vi "CalibratedGratingv1 (obsolite).vi"() -> ()   [LabVIEW 2019]
panel:
  in  "Calibration constant":dbl=1889.0 format="%#_13g"
  in  "Laser:":u16(ring) items=["800nm  "]
  out "Position on spectrometer (pixels):":dbl
  in  "?":bool
  out "Highest Harmonic:":dbl
  out "Lowest Harmonic:":dbl
  out "Beta2 (deg):":dbl
  out "Beta1 (deg):":dbl
  in  "Grating:":u16(ring) items=["Shimadzu 30-006  "]
  out "Anglular position of peak (deg):":dbl
  in  "Harmonic":dbl min=10.0 max=40.0
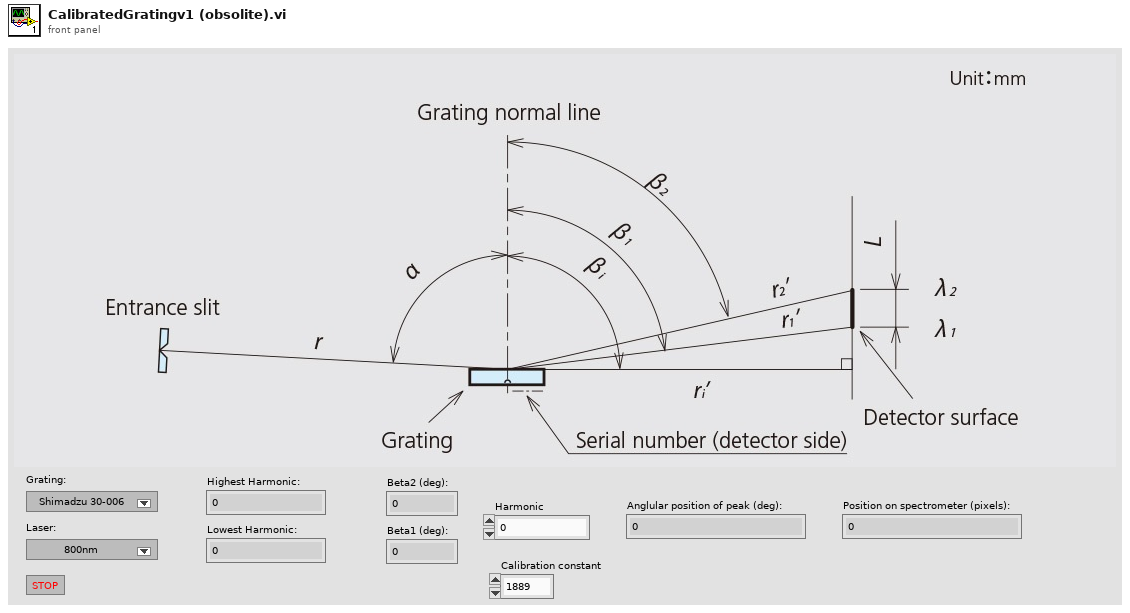
[diagram p1: front panel]
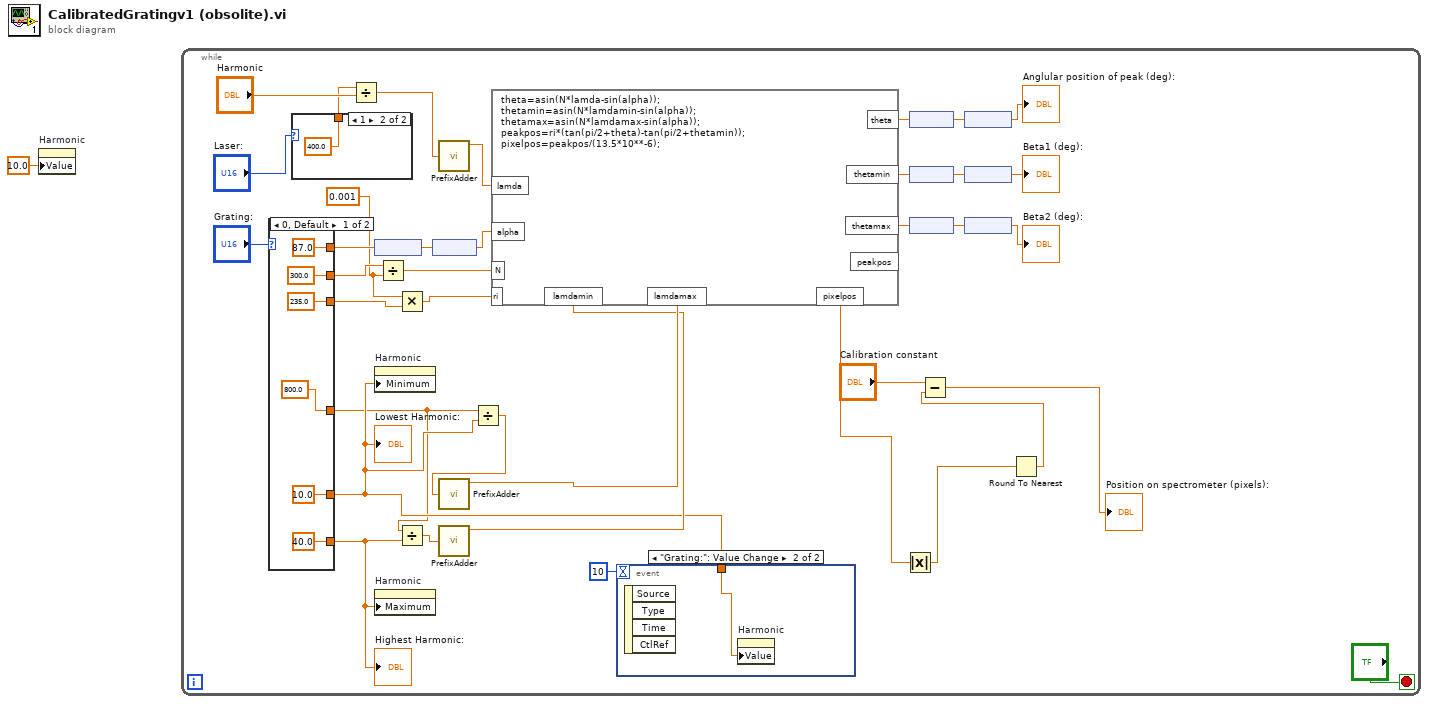
[diagram p0: block diagram]
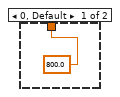
[diagram p2: hidden frame]
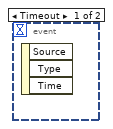
[diagram p3: hidden frame]
diagram:
  n1 = property on="Harmonic" class="DigNum (strict)"("Value"=10.0 ("Wavelegnth (nm)")) -> ()  [unwired: 2 in, 2 out]
  n2 = while {
    stop <- "?" stop-if-true
    w19 = 0.001 ("y")
    n3 = case shown="0, Default" "Grating:" {
      tunnel: [300.0 _] -> w35
      tunnel: [87.0 _] -> w34
      tunnel: [10.0 _] -> w8
      tunnel: [40.0 _] -> w9
      tunnel: [235.0 _] -> w21
      tunnel: [800.0 _] -> w2
      frame 0, Default {
      }
      frame 1 {
      }
    }
    "Lowest Harmonic:" <- w8
    "Highest Harmonic:" <- w9
    n4 = case shown="1" "Laser:" {
      tunnel: [800.0 400.0] -> w3
      frame 0, Default {
      }
      frame 1 {
      }
    }
    n5 = Divide(x=w3, y="Harmonic") -> (x/y=w16:dbl)
    n6 = node(w34) -> (w33:dbl[unit])
    n7 = property on="Harmonic" class="DigNum (strict)"("Minimum"=w8) -> ()  [unwired: 2 in, 2 out]
    n8 = property on="Harmonic" class="DigNum (strict)"("Maximum"=w9) -> ()  [unwired: 2 in, 2 out]
    n9 = Divide(x=w35, y=w19) -> (x/y=w36:dbl)
    n10 = Multiply(x=w19, y=w21) -> (x*y=w20:dbl)
    n11 = Divide(x=w2, y=w9) -> (x/y=w11:dbl)
    n12 = node(w33) -> (w32:dbl)
    n13 = call "PrefixAdder.vi"("No prefix"=w16) -> ("Nano"=w37:dbl)  [unwired: 3 out]
    n14 = call "PrefixAdder.vi"("No prefix"=w11) -> ("Nano"=w12:dbl)  [unwired: 3 out]
    n15 = Divide(x=w2, y=w8) -> (x/y=w10:dbl)
    n16 = call "PrefixAdder.vi"("No prefix"=w10) -> ("Nano"=w13:dbl)  [unwired: 3 out]
    n17 = formula code="theta=asin(N*lamda-sin(alpha));\nthetamin=asin(N*lamdamin-sin(alpha));\nthetamax=asin(N*lamdamax-sin(alpha));\npeakpos=ri*(tan(pi/2+theta)-tan(pi/2+thetamin));\npixelpos=peakpos/(13.5*10**-6);"("lamda"=w37, "N"=w36, "alpha"=w32, "lamdamin"=w12, "lamdamax"=w13, "ri"=w20) -> ("theta"=w22:dbl, "thetamin"=w26:dbl, "thetamax"=w27:dbl, "pixelpos"=w14:dbl)  [unwired: 1 out]
    n18 = event shown="[1] \"Grating:\": Value Change" {
      selector: _ -> [_ _]
      dyn-events: _ -> [_ _]
      timeout: 10 -> [_ _]
      tunnel: w8 -> [_ w41]
      event Timeout {
        n19 = event-data() -> ()  [unwired: 1 in, 3 out]
      }
      event "Grating:": Value Change {
        n20 = event-data() -> ()  [unwired: 1 in, 4 out]
        n21 = property on="Harmonic" class="DigNum (strict)"("Value"=w41) -> ()  [unwired: 2 in, 2 out]
      }
    }
    n22 = Absolute Value(x=w14) -> (abs(x)=w5:dbl)
    n23 = node(w22) -> (w31:dbl[unit])
    n24 = node(w26) -> (w29:dbl[unit])
    n25 = node(w27) -> (w28:dbl[unit])
    n26 = node(w31) -> (→"Anglular position of peak (deg):":dbl)
    n27 = node(w29) -> (→"Beta1 (deg):":dbl)
    n28 = node(w28) -> (→"Beta2 (deg):":dbl)
    n29 = Round To Nearest(number=w5) -> (nearest integer value=w4:dbl)
    n30 = Subtract(x="Calibration constant", y=w4) -> (x-y=→"Position on spectrometer (pixels):":dbl)
  }
